vi "SendString.vi"(8 "error in (no error)":errorcluster, 10 "data in":string, 11 "TCP Connection in":refnum<class "TCP Connection.lvclass">) -> (0 "error out":errorcluster, 2 "bytes written":i32, 3 "TCP Connection out":refnum<class "TCP Connection.lvclass">)   [LabVIEW 2011, in "TCP Connection.lvclass"]
doc: "Sends the input string to the instantiated TCP Connection."
uses:
  TCP Connection.lvclass
  TCP Connection.lvclass/TCP Connection.ctl
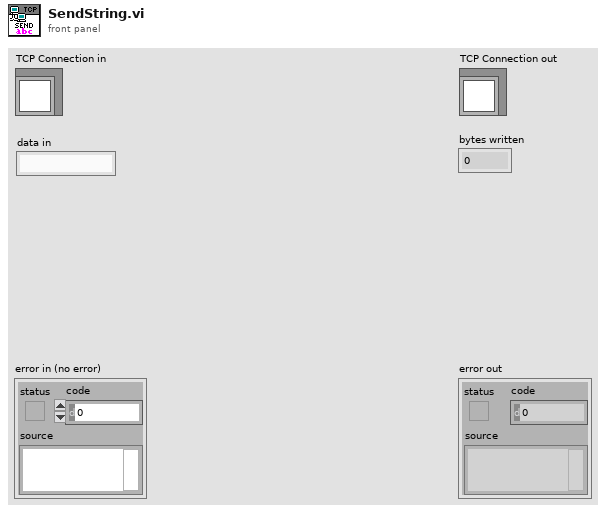
[diagram p1: front panel]
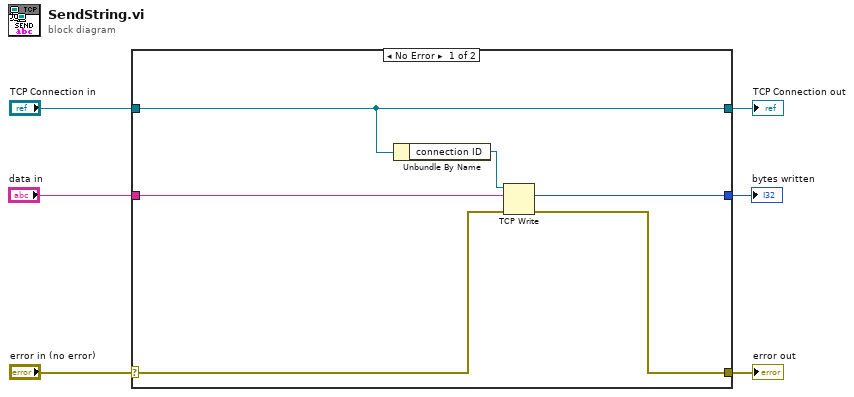
[diagram p0: block diagram]
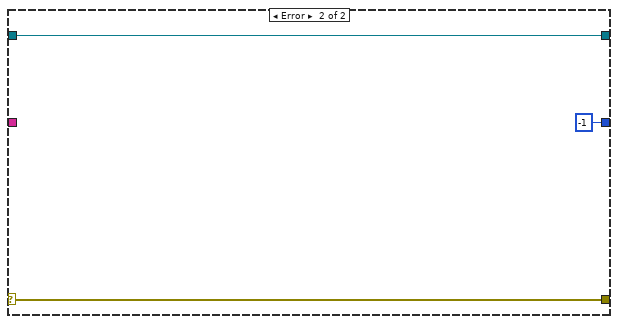
[diagram p2: hidden frame]
diagram:
  n1 = case shown="No Error" "error in (no error)" {
    selector: "error in (no error)" -> [w10 w15]
    tunnel: [w9 w15] -> w5
    tunnel: [w12 w14] -> w3
    tunnel: "TCP Connection in" -> [w12 w14]
    tunnel: [w8 -1 ("bytes written")] -> w2
    tunnel: "data in" -> [w7 _]
    frame No Error {
      n2 = Unbundle By Name(w12) -> ("connection ID"=w11:refnum<k5>)
      n3 = TCP Write(connection ID=w11, data in=w7, error in (no error)=w10) -> (bytes written=w8:i32, error out=w9:errorcluster)  [unwired: 1 in, 1 out]
    }
    frame Error {
    }
  }
  "error out" <- w5
  "TCP Connection out" <- w3
  "bytes written" <- w2
